vi "ConvertItemListToFormatElements.vi"(11 "Item List":string) -> (3 "Format Elements":T1[](array[typedef]))   [LabVIEW 2012, in "Keithley-6485.lvlib"]
uses:
  Keithley-6485.lvlib
  Public/Controls/FormatElement.ctl
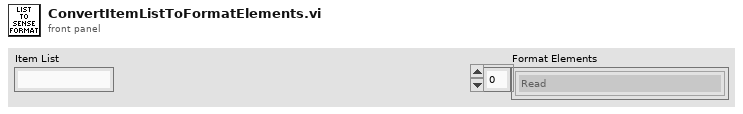
[diagram p1: front panel]
types:
  T1 = typedef "Keithley-6485.lvlib/FormatElement.ctl" = enum16{"Read", "Unit", "Time", "Status"}
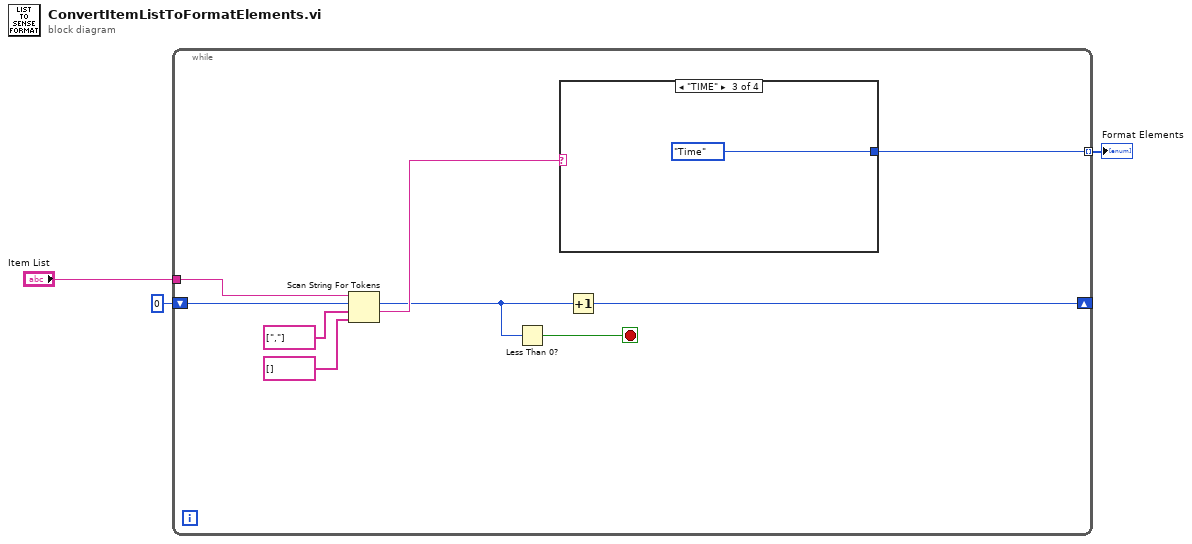
[diagram p0: block diagram]
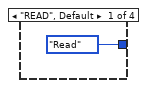
[diagram p2: hidden frame]
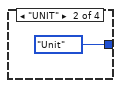
[diagram p3: hidden frame]
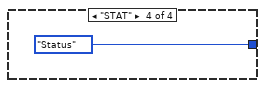
[diagram p4: hidden frame]
diagram:
  n1 = while {
    shift-right: [w4] -> _
    shift-left: 0 ("offset past token") -> [w12]
    tunnel: [w10] -> w2 mode=indexing
    tunnel: "Item List" -> [w7]
    stop <- w6 stop-if-true
    n2 = Scan String For Tokens(6:string[] [] ("delimiters (\\s,\\t,\\r,\\n)"), 7:string[] [","] ("delimiters (\\s,\\t,\\r,\\n)"), 8:w12, 9:w7) -> (1:w11:string, 2:w5:i32)  [unwired: 2 in, 2 out]
    n3 = Less Than 0?(x=w5) -> (x < 0?=w6:bool)
    n4 = case shown="\"TIME\"" w11 {
      tunnel: [FormatElement."Read" ("Format Sense Element") FormatElement."Unit" ("Format Sense Element") FormatElement."Time" ("Format Sense Element") FormatElement."Status" ("Format Sense Element")] -> w10
      frame "READ", Default {
      }
      frame "UNIT" {
      }
      frame "TIME" {
      }
      frame "STAT" {
      }
    }
    n5 = Increment(x=w5) -> (x+1=w4:i32)
  }
  "Format Elements" <- w2
